vi "GetBroadcast.vi"(7 "ModuleID":i32, 8 "error in (no error)":errorcluster, 11 "ModuleType":T1) -> (0 "error out":errorcluster, 1 "Data":variant, 2 "Recvd":string)   [LabVIEW 2014, in "BusController.lvlib"]
uses:
  BusController.lvlib
  ModuleType.ctl
  <vilib>/Utility/error.llb/Error Cluster From Error Code.vi
  <vilib>/ErrorRing/Error Ring.xnode
  Modules/PmuImpairModule/PmuImpairModule.lvlib
  Modules/EventModule/EventModule.lvlib
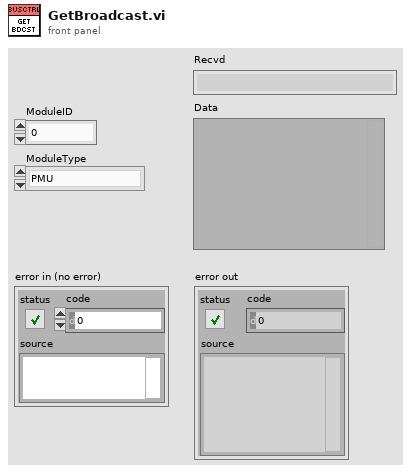
[diagram p1: front panel]
types:
  T1 = typedef "BusController.lvlib/ModuleType.ctl" = enum16{"PMU", "Event", "Network", "Flag", "App"}
  T2 = typedef "PmuImpairModule.lvlib/clBroadcastEvents.ctl" = cluster{"DidInit":refnum<user-event>, "StatusUpdate":refnum<user-event>, "ErrorReport":refnum<user-event>, "DidStop":refnum<user-event>, "ImpairConfig":refnum<user-event>, "ImpairParams":refnum<user-event>, "ImpairReports":refnum<user-event>, "PathToPlugin":refnum<user-event>, "BusNumber":refnum<user-event>}
  T3 = typedef "EventModule.lvlib/clBroadcastEvents.ctl" = cluster{"DidInit":refnum<user-event>, "StatusUpdate":refnum<user-event>, "ErrorReport":refnum<user-event>, "DidStop":refnum<user-event>, "ReadEvtConfig":refnum<user-event>, "ReadTimeArray":refnum<user-event>, "ReadEvtParams":refnum<user-event>, "GetEvtReportArray":refnum<user-event>, "ReadPathToPlugin":refnum<user-event>, "GetEvtSignal":refnum<user-event>, "ReadBusNumber":refnum<user-event>}
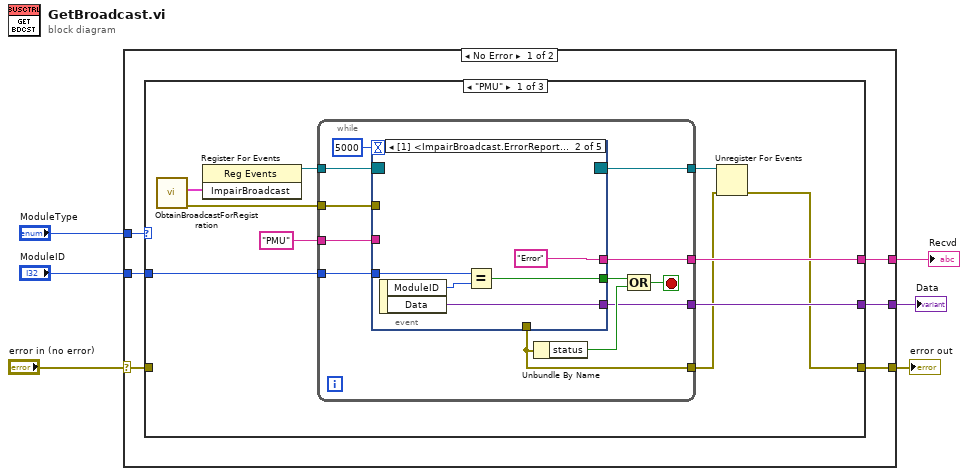
[diagram p0: block diagram]
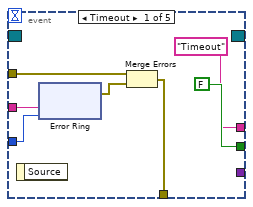
[diagram p2: hidden frame]
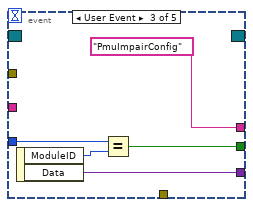
[diagram p3: hidden frame]
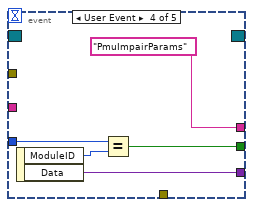
[diagram p4: hidden frame]
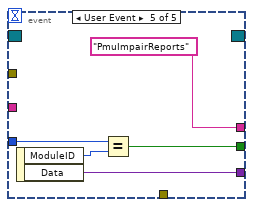
[diagram p5: hidden frame]
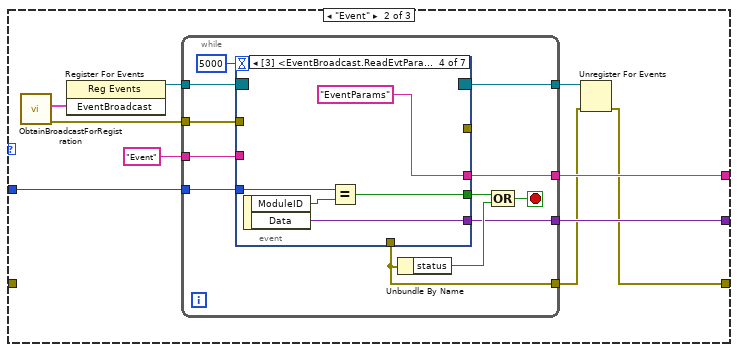
[diagram p6: hidden frame]
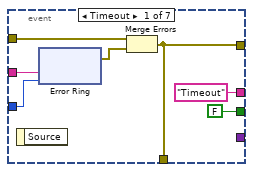
[diagram p7: hidden frame]
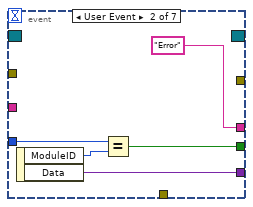
[diagram p8: hidden frame]
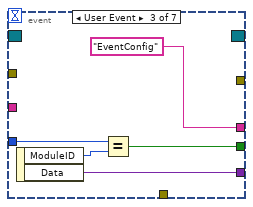
[diagram p9: hidden frame]
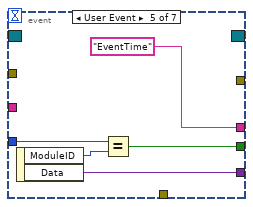
[diagram p10: hidden frame]
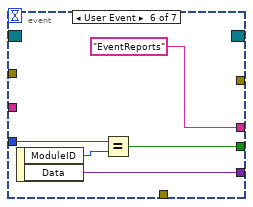
[diagram p11: hidden frame]
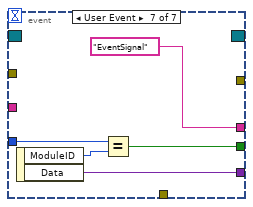
[diagram p12: hidden frame]
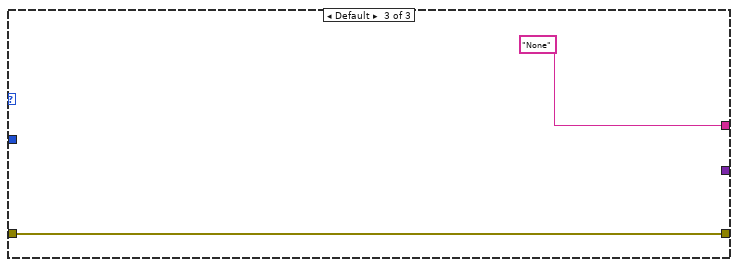
[diagram p13: hidden frame]
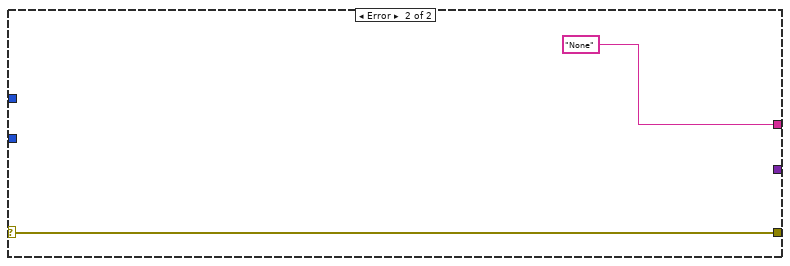
[diagram p14: hidden frame]
diagram:
  n1 = case shown="No Error" "error in (no error)" {
    selector: "error in (no error)" -> [w9 w140]
    tunnel: [w11 w140] -> w5
    tunnel: [w10 "None"] -> w4
    tunnel: "ModuleType" -> [w12 _]
    tunnel: "ModuleID" -> [w8 _]
    tunnel: [w7 _] -> w1
    frame No Error {
      n2 = case shown="\"PMU\"" w12 {
        tunnel: [w13 w71 w138] -> w11
        tunnel: [w20 w76 "None"] -> w10
        tunnel: w9 -> [_ _ w138]
        tunnel: w8 -> [w19 w75 _]
        tunnel: [w18 w74 _] -> w7
        frame "PMU" {
          n3 = call "ObtainBroadcastForRegistration.vi"() -> ("error out"=w21:errorcluster, "ImpairBroadcast"=w14:T2)  [unwired: 10 in]
          n4 = register-events(w14) -> (reference out=w22:refnum<event-registration>)  [unwired: 2 in, 1 out]
          n5 = while {
            tunnel: w22 -> [w33]
            tunnel: w21 -> [w32]
            tunnel: [w31] -> w15
            tunnel: [w27] -> w20
            tunnel: w19 -> [w26]
            tunnel: [w25] -> w18
            tunnel: "PMU" -> [w24]
            tunnel: [w23] -> w16
            stop <- w28 stop-if-true
            n6 = event shown="[1] <ImpairBroadcast.ErrorReport>: User Event" {
              selector: w33 -> [_ _ _ _ _]
              dyn-events: [_ _ _ _ _] -> w23
              timeout: 5000 -> [_ _ _ _ _]
              tunnel: w32 -> [w41 _ _ _ _]
              tunnel: w24 -> [w39 _ _ _ _]
              tunnel: [w38 _ _ _ _] -> w31
              tunnel: [FALSE w51 w56 w61 w66] -> w30
              tunnel: ["Timeout" "Error" "PmuImpairConfig" "PmuImpairParams" "PmuImpairReports"] -> w27
              tunnel: w26 -> [w35 w52 w57 w62 w67]
              tunnel: [_ w50 w55 w60 w65] -> w25
              event Timeout {
                n7 = event-data() -> ()  [unwired: 1 in, 1 out]
                n8 = xnode "Error Ring"("parameter 0"=w39, "parameter 1"=w35) -> ("error out"=w40:errorcluster)
                n9 = Merge Errors(w41, w40) -> (w38:errorcluster)
              }
              event User Event {
                n10 = event-data() -> ("ModuleID"=w53:i32, "Data"=w50:variant)  [unwired: 1 in]
                n11 = Equal?(x=w52, y=w53) -> (x = y?=w51:bool)
              }
              event User Event {
                n12 = event-data() -> ("ModuleID"=w58:i32, "Data"=w55:variant)  [unwired: 1 in]
                n13 = Equal?(x=w57, y=w58) -> (x = y?=w56:bool)
              }
              event User Event {
                n14 = event-data() -> ("ModuleID"=w63:i32, "Data"=w60:variant)  [unwired: 1 in]
                n15 = Equal?(x=w62, y=w63) -> (x = y?=w61:bool)
              }
              event User Event {
                n16 = event-data() -> ("ModuleID"=w68:i32, "Data"=w65:variant)  [unwired: 1 in]
                n17 = Equal?(x=w67, y=w68) -> (x = y?=w66:bool)
              }
            }
            n18 = Unbundle By Name(w31) -> ("status"=w29:bool)
            n19 = Compound Arithmetic op=OR(w30, w29) -> (w28:bool)
          }
          n20 = Unregister For Events(event registration refnum=w16, error in=w15) -> (error out=w13:errorcluster)
        }
        frame "Event" {
          n21 = call "ObtainBroadcastForRegistration.vi"() -> ("error out"=w77:errorcluster, "EventBroadcast"=w79:T3)  [unwired: 10 in]
          n22 = register-events(w79) -> (reference out=w78:refnum<event-registration>)  [unwired: 2 in, 1 out]
          n23 = while {
            tunnel: w78 -> [w82]
            tunnel: w77 -> [w90]
            tunnel: [w80] -> w70
            tunnel: [w86] -> w76
            tunnel: w75 -> [w85]
            tunnel: [w84] -> w74
            tunnel: "Event" -> [w83]
            tunnel: [w81] -> w72
            stop <- w87 stop-if-true
            n24 = event shown="[3] <EventBroadcast.ReadEvtParams>: User Event" {
              selector: w82 -> [_ _ _ _ _ _ _]
              dyn-events: [_ _ _ _ _ _ _] -> w81
              timeout: 5000 -> [_ _ _ _ _ _ _]
              tunnel: w90 -> [w98 _ _ _ _ _ _]
              tunnel: w83 -> [w96 _ _ _ _ _ _]
              tunnel: [w92 _ _ _ _ _ _] -> w80
              tunnel: [FALSE w108 w113 w118 w123 w128 w133] -> w89
              tunnel: ["Timeout" "Error" "EventConfig" "EventParams" "EventTime" "EventReports" "EventSignal"] -> w86
              tunnel: w85 -> [w93 w109 w114 w119 w124 w129 w134]
              tunnel: [_ w107 w112 w117 w122 w127 w132] -> w84
              tunnel: [w92 _ _ _ _ _ _] -> _
              event Timeout {
                n25 = event-data() -> ()  [unwired: 1 in, 1 out]
                n26 = xnode "Error Ring"("parameter 0"=w96, "parameter 1"=w93) -> ("error out"=w97:errorcluster)
                n27 = Merge Errors(w98, w97) -> (w92:errorcluster)
              }
              event User Event {
                n28 = event-data() -> ("ModuleID"=w110:i32, "Data"=w107:variant)  [unwired: 1 in]
                n29 = Equal?(x=w109, y=w110) -> (x = y?=w108:bool)
              }
              event User Event {
                n30 = event-data() -> ("ModuleID"=w115:i32, "Data"=w112:variant)  [unwired: 1 in]
                n31 = Equal?(x=w114, y=w115) -> (x = y?=w113:bool)
              }
              event User Event {
                n32 = event-data() -> ("ModuleID"=w120:i32, "Data"=w117:variant)  [unwired: 1 in]
                n33 = Equal?(x=w119, y=w120) -> (x = y?=w118:bool)
              }
              event User Event {
                n34 = event-data() -> ("ModuleID"=w125:i32, "Data"=w122:variant)  [unwired: 1 in]
                n35 = Equal?(x=w124, y=w125) -> (x = y?=w123:bool)
              }
              event User Event {
                n36 = event-data() -> ("ModuleID"=w130:i32, "Data"=w127:variant)  [unwired: 1 in]
                n37 = Equal?(x=w129, y=w130) -> (x = y?=w128:bool)
              }
              event User Event {
                n38 = event-data() -> ("ModuleID"=w135:i32, "Data"=w132:variant)  [unwired: 1 in]
                n39 = Equal?(x=w134, y=w135) -> (x = y?=w133:bool)
              }
            }
            n40 = Unbundle By Name(w80) -> ("status"=w88:bool)
            n41 = Compound Arithmetic op=OR(w89, w88) -> (w87:bool)
          }
          n42 = Unregister For Events(event registration refnum=w72, error in=w70) -> (error out=w71:errorcluster)
        }
        frame Default {
        }
      }
    }
    frame Error {
    }
  }
  "error out" <- w5
  "Recvd" <- w4
  "Data" <- w1
